vi "Actor Teardown Core.vi"(7 "Actor in":refnum<class "Actor.lvclass">, 11 "Destroying Self Actor State in":refnum<class "Destroying Self Actor State.lvclass">) -> (2 "Teardown?":bool, 5 "Actor out":refnum<class "Actor.lvclass">)   [LabVIEW 2021, in "jettl.lvlib" / "Destroying Self Actor State.lvclass"]
uses:
  Destroying Self Actor State.lvclass
  Actor/Actor.lvclass
  Msgs/Actor Last Ack/Actor Last Ack Msg Strategy/Actor Last Ack Msg Strategy.lvclass
  C:/git/jettl/src/jettl/Msg Strategy/Msg Strategy.lvclass
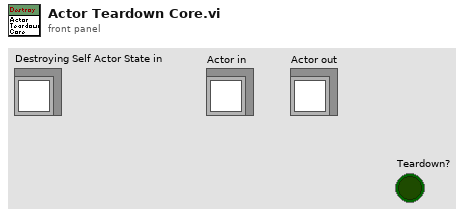
[diagram p1: front panel]
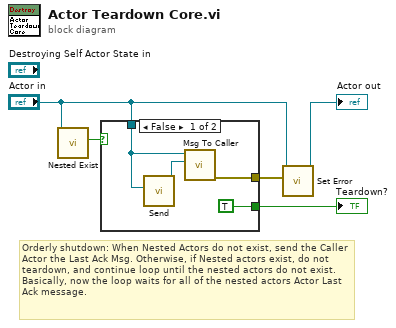
[diagram p0: block diagram]
diagram:
  # "Orderly shutdown: When Nested Actors do not exist, send the Caller Actor the Last Ack Msg. Otherwise, if Nested actors exist, do not teardown, and continue loop until the nested actors do not exist. Basically, now the loop waits for all of the nested actors Actor Last Ack message."
  n1 = call-dynamic "Nested Exist.vi"("Actor in"="Actor in") -> ("Nested Exist?"=w4:bool)  [unwired: 10 in]
  n2 = case shown="False" w4 {
    tunnel: "Actor in" -> [w8 _]
    tunnel: [TRUE ("Destroyed?") _] -> w5
    tunnel: [w6 _] -> w2
    frame False {
      n3 = call "Send.vi"("Nested Actor"=w8) -> ("Actor Last Ack Msg Strategy out"=w7:refnum<class "Actor Last Ack Msg Strategy.lvclass">)  [unwired: 10 in]
      n4 = call-dynamic "Msg To Caller.vi"("Msg"=w7, "Actor in"=w8) -> ("error out"=w6:errorcluster)  [unwired: 9 in]
    }
    frame True {
    }
  }
  "Teardown?" <- w5
  n5 = call-dynamic "Set Error.vi"("Error"=w2, "Actor in"="Actor in") -> ("Actor out"=→"Actor out":refnum<class "Actor.lvclass">)  [unwired: 9 in]
